vi "Launcher.vi"   [LabVIEW 2015]
uses:
  <vilib>/ActorFramework/Actor/Actor.lvclass
  Calling Actor/Calling Actor.lvclass
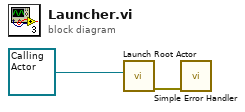
[diagram p0: block diagram]
diagram:
  n1 = call <vilib>:"Launch Root Actor.vi"("Actor"=refnum<class "Calling Actor.lvclass"> refnum ("Calling Actor.lvlib:Calling Actor.lvclass")) -> ("error out"=w2:errorcluster)  [unwired: 9 in, 1 out]
  n2 = call <vilib>:"Simple Error Handler.vi"("error in (no error)"=w2) -> ()  [unwired: 4 in, 5 out]
